vi "Logging Data.vi"(11 "Drive Loop Cluster":T3) -> (3 "Logging Data":T1)   [LabVIEW 2015]
uses:
  <userlib>/836-Library/Drive/Drive Code/Drive Code Support/Drive Code Bundle.ctl
  <userlib>/836-Library/Drive/Drive Code/Drive Code Support/Sensor Cluster.ctl
  <userlib>/836-Library/Drive/Drive Code/Drive Code Support/Camera Cluster.ctl
  <userlib>/836-Library/Drive/Drive Code/Drive Code Support/Drive Code Notifier.ctl
  <userlib>/836-Library/Drive/Drive Code/Drive Code Support/Drive Code Command.ctl
  <userlib>/836-Library/Drive/Drive Code/Logging Data.ctl
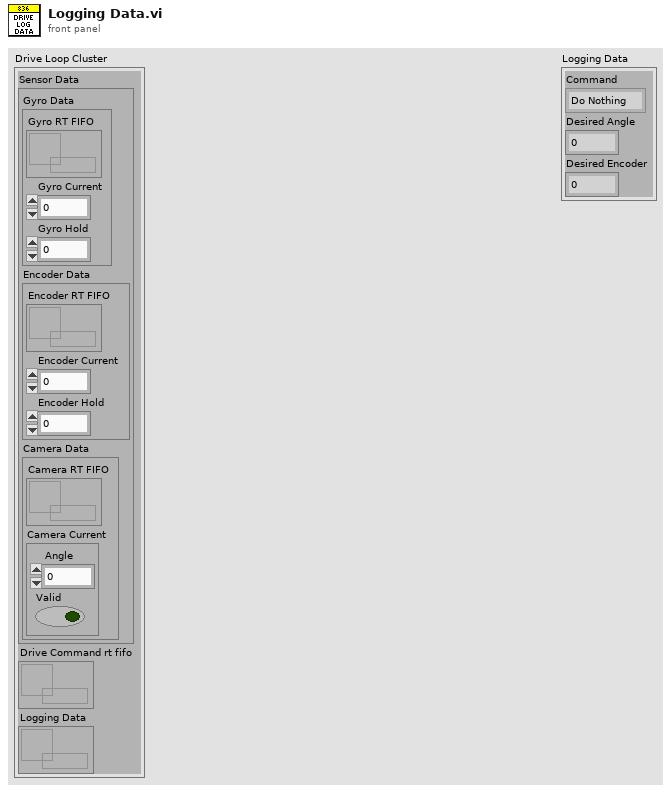
[diagram p1: front panel]
types:
  T1 = typedef "Logging Data.ctl" = cluster{"Command":T2, "Desired Angle":dbl, "Desired Encoder":dbl}
  T2 = typedef "Drive Code Command.ctl" = enum16{"Do Nothing", "Manual", "Drive Continuous", "Turn", "Drive Distance", "Hold Position", "Hold Yaw", "Follow Camera", "Turn to Camera"}
  T3 = typedef "Drive Code Bundle.ctl" = cluster{"Sensor Data":T4, "Drive Command rt fifo":refnum<k33>, "Logging Data":refnum<k33>}
  T4 = typedef "Sensor Cluster.ctl" = cluster{"Gyro Data":cluster{"Gyro RT FIFO":refnum<k33>, "Gyro Current":dbl, "Gyro Hold":dbl}, "Encoder Data":cluster{"Encoder RT FIFO":refnum<k33>, "Encoder Current":dbl, "Encoder Hold":dbl}, "Camera Data":cluster{"Camera RT FIFO":refnum<k33>, "Camera Current":T5}}
  T5 = typedef "Camera Cluster.ctl" = cluster{" Angle":dbl, "Valid":bool}
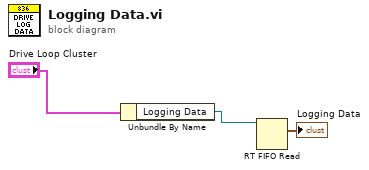
[diagram p0: block diagram]
diagram:
  n1 = Unbundle By Name("Drive Loop Cluster") -> ("Logging Data"=w2:refnum<k33>)
  n2 = RT FIFO Read(0:w2) -> (9:→"Logging Data":T1)  [unwired: 3 in, 4 out]
